vi "op_biti_v4.vi"() -> ()   [LabVIEW 2009]
panel:
  out "Array":bool[](array[boolean])=[TRUE, FALSE, FALSE, TRUE, TRUE, FALSE, FALSE, TRUE]
  out "Boolean":bool=TRUE
  in  "Boolean":bool=TRUE
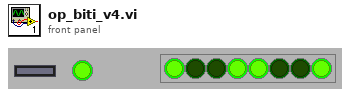
[diagram p1: front panel]
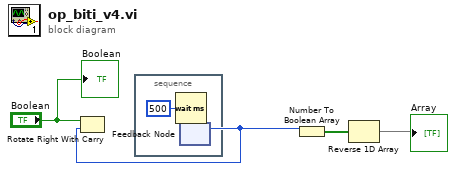
[diagram p0: block diagram]
diagram:
  n1 = stacked-sequence {
    frame #0 {
      n2 = Wait (ms)(milliseconds to wait=500) -> ()  [unwired: 1 out]
    }
  }
  n3 = feedback #1() -> (w1:u8)  [unwired: 1 in]
  n4 = Rotate Right With Carry(2:w1, 3:"Boolean") -> (0:w5:u8)  [unwired: 1 out]
  n5 = Number To Boolean Array(number=w1) -> (Boolean array=w3:bool[])
  n6 = Reverse 1D Array(array=w3) -> (reversed array=→"Array":bool[])
  "Boolean" <- "Boolean"
